vi "DDS Initialize.vi"(8 "error in (no error)":errorcluster, 11 "DDS ref in":T1={"NI USB-8451 device reference"="", "DIO port"=0, "Serial Clock Rate [kHz]"=1000}) -> (0 "error out":errorcluster, 3 "DDS ref out":T1={"NI USB-8451 device reference"="", "DIO port"=0, "Serial Clock Rate [kHz]"=1000})   [LabVIEW 2013, in "DDS.lvlib"]
doc: "For each of the four AD9910 chips in the DDS box:\n\nResets and initilizes the AD9910 chip on the specified port. Sets the TTL lines to output low. Configures 3-wire (SPI) communication. Disables the clock divider. An external reference clock is expected (the PLL is not enabled)."
uses:
  DDS.lvlib
  Controls/DDS Box Device Reference.ctl
  <vilib>/ni845x/ni845x.llb/ni845xControl.ctl
  <vilib>/ni845x/ni845x.llb/ni845xDioLineConfiguration.ctl
  <vilib>/ni845x/ni845x.llb/ni845xDioLineWriteValue.ctl
  Controls/DDS CS pins.ctl
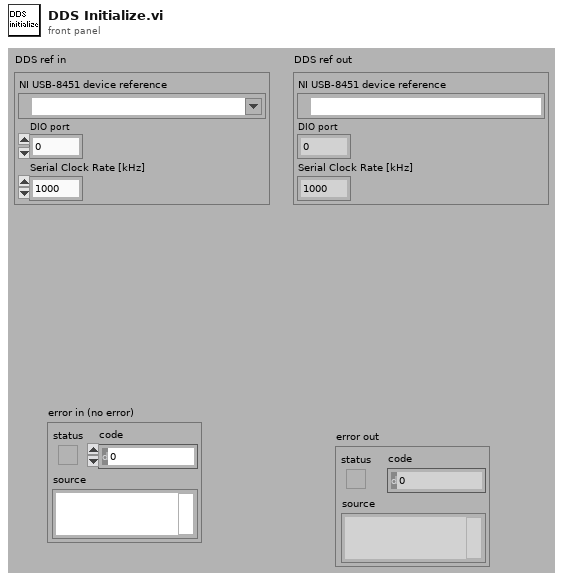
[diagram p1: front panel]
types:
  T1 = typedef "DDS.lvlib/DDS Box Device Reference.ctl" = cluster{"NI USB-8451 device reference":T2, "DIO port":u8, "Serial Clock Rate [kHz]":u16}
  T2 = typedef "ni845xControl.ctl" = refnum<k21>
  T3 = typedef "DDS.lvlib/DDS CS pins.ctl" = enum8{"IO reset", "Ch. 4 CS", "Ch. 3 CS", "Ch. 2 CS", "Ch. 1 CS"}
  T4 = typedef "ni845xDioLineWriteValue.ctl" = i32
  T5 = typedef "ni845xDioLineConfiguration.ctl" = i32
  T6 = typedef "ni845xSpiScriptControl.ctl" = refnum<k20>
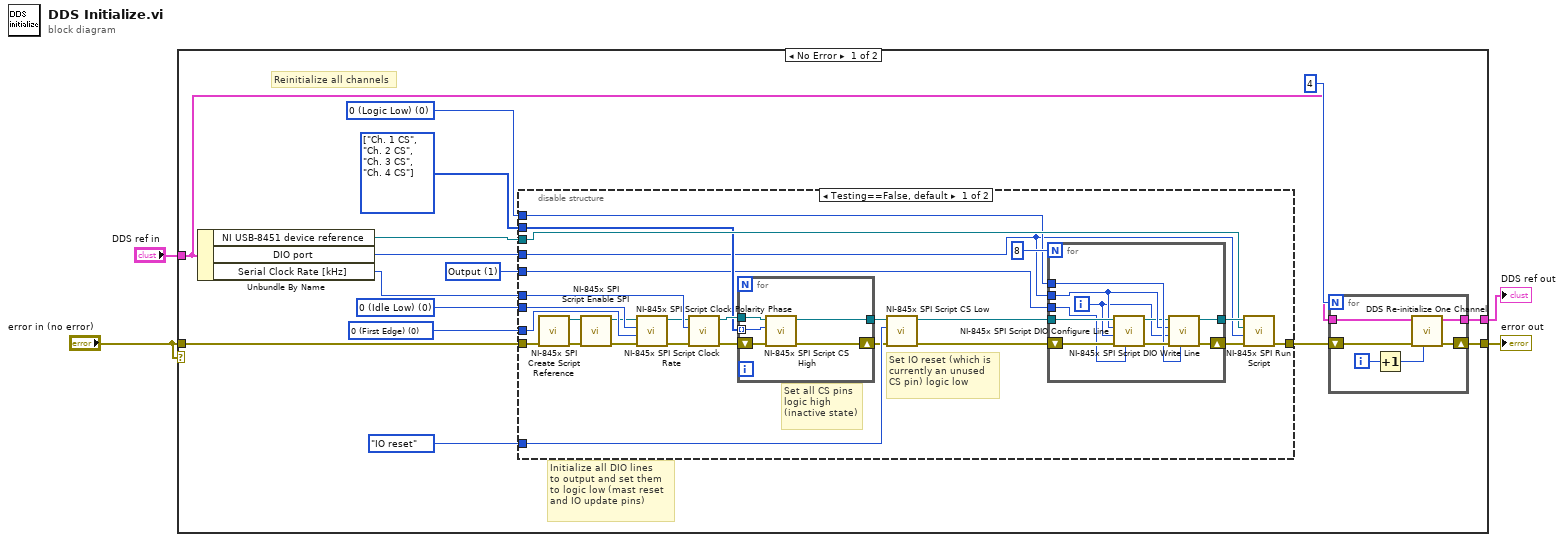
[diagram p0: block diagram]
diagram:
  n1 = case shown="No Error" "error in (no error)" {
    tunnel: "error in (no error)" -> [w17 w68]
    tunnel: "DDS ref in" -> [w5 w69]
    tunnel: [w14 w69] -> w2
    tunnel: [w15 w68] -> w1
    frame No Error {
      w8 = T3[] [enum."Ch. 1 CS", enum."Ch. 2 CS", enum."Ch. 3 CS", enum."Ch. 4 CS"] items=["IO reset", "Ch. 4 CS", "Ch. 3 CS", "Ch. 2 CS", "Ch. 1 CS"]
      w6 = T4 0 items=["0 (Logic Low)", "1 (Logic High)"] ("write value")
      w7 = T5 1 items=["Input", "Output"] ("configuration (input)")
      w19 = 0 items=["0 (First Edge)", "1 (Second Edge)"] ("clock phase (0)")
      w18 = 0 items=["0 (Idle Low)", "1 (Idle High)"] ("clock polarity (0)")
      # "Reinitialize all channels"
      # "Initialize all DIO lines\nto output and set them\nto logic low (mast reset\nand IO update pins)"
      n2 = Unbundle By Name(w5) -> ("NI USB-8451 device reference"=w10:T2, "DIO port"=w11:u8, "Serial Clock Rate [kHz]"=w16:u16)
      n3 = disable-structure shown="Testing==False, default" {
        disable-tunnel: w19 -> [w45 _]
        disable-tunnel: w18 -> [w44 _]
        disable-tunnel: w17 -> [w43 w61]
        disable-tunnel: w16 -> [w42 _]
        disable-tunnel: [w35 w61] -> w13
        disable-tunnel: w11 -> [w20 _]
        disable-tunnel: w10 -> [w29 _]
        disable-tunnel: DDS_CS_pins."IO reset" ("DDS CS pins") -> [w28 _]
        disable-tunnel: w8 -> [w27 _]
        disable-tunnel: w7 -> [w22 _]
        disable-tunnel: w6 -> [w21 _]
        frame condition #0 (active) {
          # "Set IO reset (which is\ncurrently an unused\nCS pin) logic low"
          # "Set all CS pins\nlogic high\n(inactive state)"
          n4 = call <vilib>:"NI-845x SPI Create Script Reference.vi"("error in (no error)"=w43) -> ("error out"=w41:errorcluster, "spi script reference"=w40:T6)  [unwired: 9 in]
          n5 = call <vilib>:"NI-845x SPI Script Enable SPI.vi"("error in (no error)"=w41, "spi script reference in"=w40) -> ("error out"=w39:errorcluster, "spi script reference out"=w38:T6)  [unwired: 8 in]
          n6 = call <vilib>:"NI-845x SPI Script Clock Polarity Phase.vi"("error in (no error)"=w39, "clock phase (0)"=w45, "clock polarity (0)"=w44, "spi script reference in"=w38) -> ("error out"=w36:errorcluster, "spi script reference out"=w37:T6)  [unwired: 6 in]
          n7 = call <vilib>:"NI-845x SPI Script Clock Rate.vi"("error in (no error)"=w36, "clock rate in kHz (1000)"=w42, "spi script reference in"=w37) -> ("error out"=w32:errorcluster, "spi script reference out"=w33:T6)  [unwired: 7 in]
          n8 = for {
            shift-right: [w47] -> w26
            shift-left: w32 -> [w49]
            tunnel: w27 -> [w46] mode=indexing
            tunnel: w33 -> [w50]
            tunnel: [w48] -> w25
            n9 = call <vilib>:"NI-845x SPI Script CS High.vi"("error in (no error)"=w49, "chip select (0)"=w46, "spi script reference in"=w50) -> ("error out"=w47:errorcluster, "spi script reference out"=w48:T6)  [unwired: 7 in]
          }
          n10 = call <vilib>:"NI-845x SPI Script CS Low.vi"("error in (no error)"=w26, "chip select (0)"=w28, "spi script reference in"=w25) -> ("error out"=w23:errorcluster, "spi script reference out"=w24:T6)  [unwired: 7 in]
          n11 = for {
            N: 8 -> [_]
            tunnel: w22 -> [w58]
            tunnel: w20 -> [w55]
            shift-right: [w52] -> w30
            shift-left: w23 -> [w60]
            tunnel: w21 -> [w56]
            tunnel: w24 -> [w59]
            tunnel: [w53] -> w31
            i -> [w51]
            n12 = call <vilib>:"NI-845x SPI Script DIO Configure Line.vi"("configuration (input)"=w58, "error in (no error)"=w60, "line number (0)"=w51, "port number (0)"=w55, "spi script reference in"=w59) -> ("error out"=w57:errorcluster, "spi script reference out"=w54:T6)  [unwired: 5 in]
            n13 = call <vilib>:"NI-845x SPI Script DIO Write Line.vi"("write value"=w56, "error in (no error)"=w57, "line number (0)"=w51, "port number (0)"=w55, "spi script reference in"=w54) -> ("error out"=w52:errorcluster, "spi script reference out"=w53:T6)  [unwired: 5 in]
          }
          n14 = call <vilib>:"NI-845x SPI Run Script.vi"("error in (no error)"=w30, "port (0)"=w20, "device reference in"=w29, "spi script reference in"=w31) -> ("error out"=w35:errorcluster)  [unwired: 5 in, 2 out]
        }
        frame condition #1 {
        }
      }
      n15 = for {
        N: 4 -> [_]
        tunnel: [w63] -> w14
        tunnel: w5 -> [w67]
        shift-right: [w64] -> w15
        shift-left: w13 -> [w65]
        i -> [w66]
        n16 = Increment(x=w66) -> (x+1=w62:i32)
        n17 = call "DDS Re-initialize One Channel.vi"("channel number (1)"=w62, "error in (no error)"=w65, "DDS ref in"=w67) -> ("error out"=w64:errorcluster, "DDS ref out"=w63:T1)  [unwired: 5 in]
      }
    }
    frame Error {
    }
  }
  "error out" <- w1
  "DDS ref out" <- w2
